vi "main.vi"() -> ()   [LabVIEW 2026]
panel:
  out "Tab Value":T1(ring)
  in  "Error In":errorcluster
  out "Value":T1(ring)
  in  "Tab Control":T1(tab)
  out "pull_indicator":bool
  in  "pull_button":bool
  in  "Commit Message":string
  out "String":string
  in  "commit _button":bool
  out "commit_indicator":bool
  out "git commit output":string
  in  "add_all_button":bool
  out "add_all_indicator":bool
  out "git add output":string
  in  "push_button":bool
  out "push_indicator":bool
  out "git push output":string
  in  "commit message":string
  in  "working directory":path=path ""
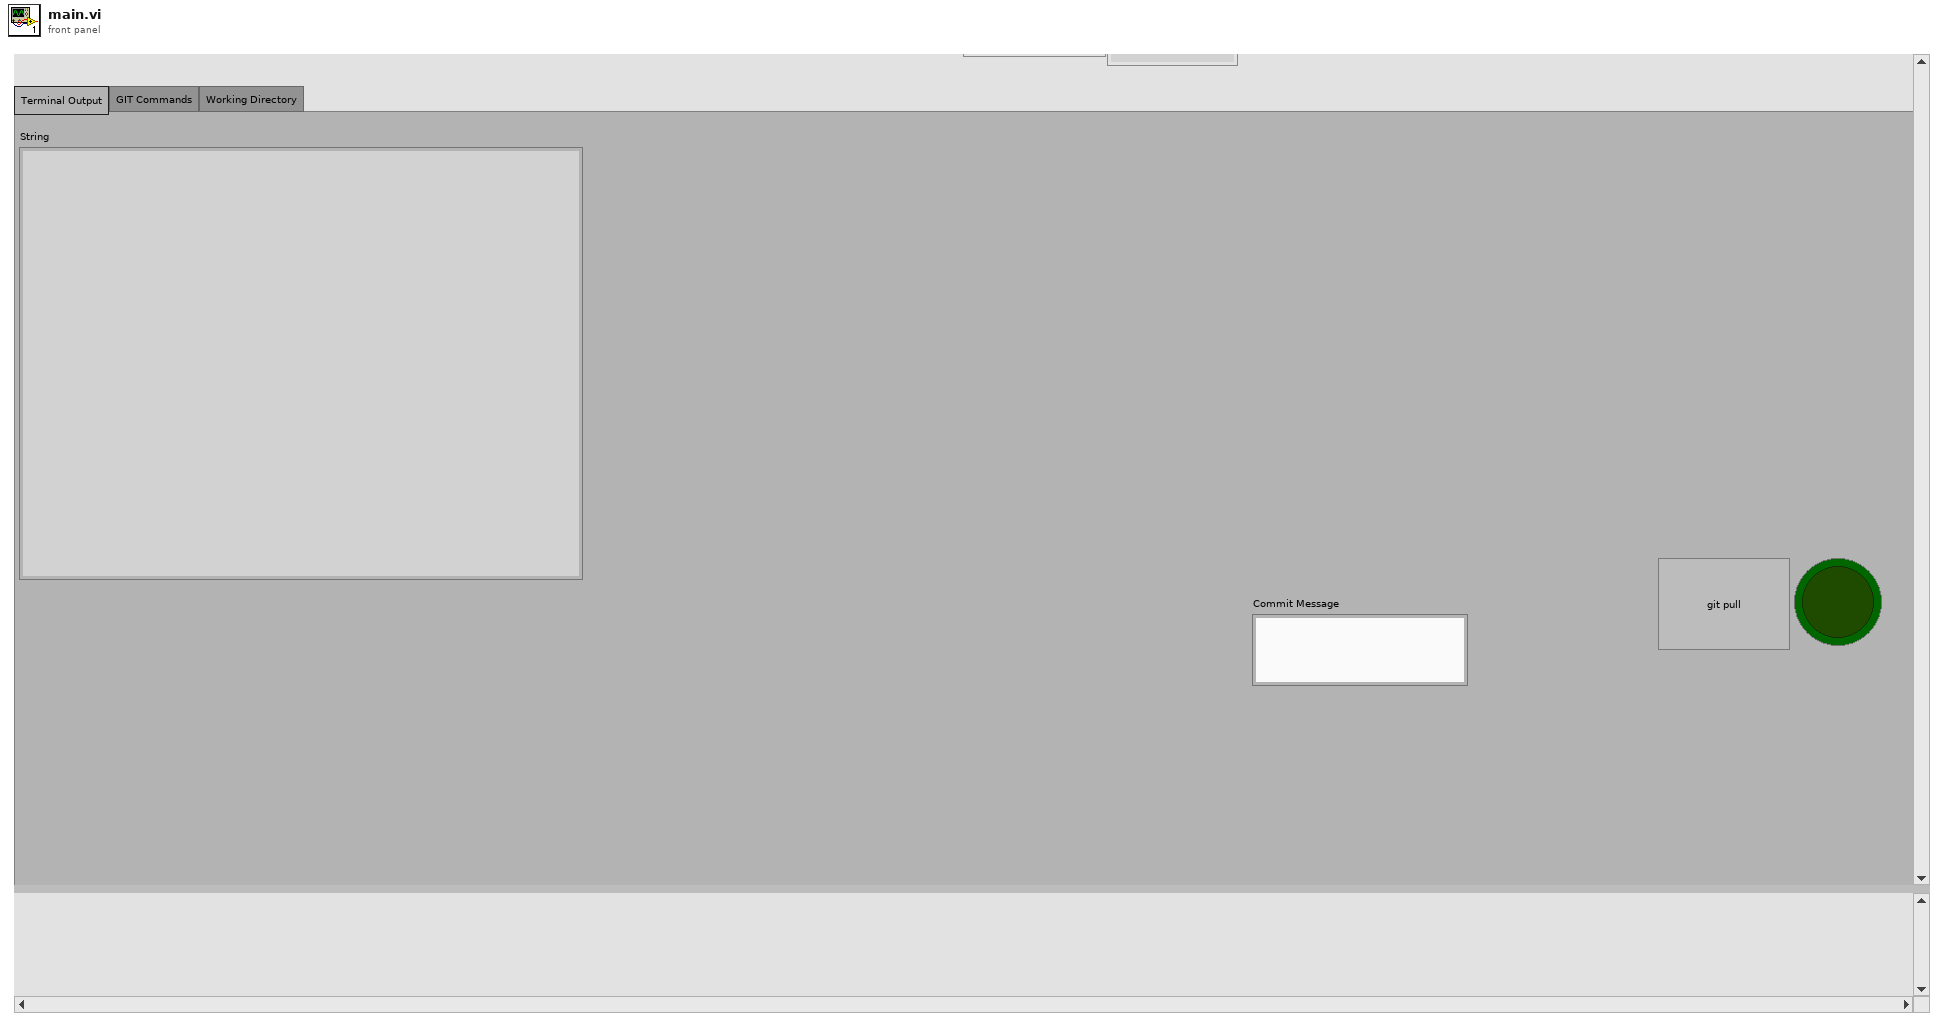
[diagram p1: front panel]
types:
  T1 = enum32{"Terminal Output", "GIT Commands", "Working Directory"}
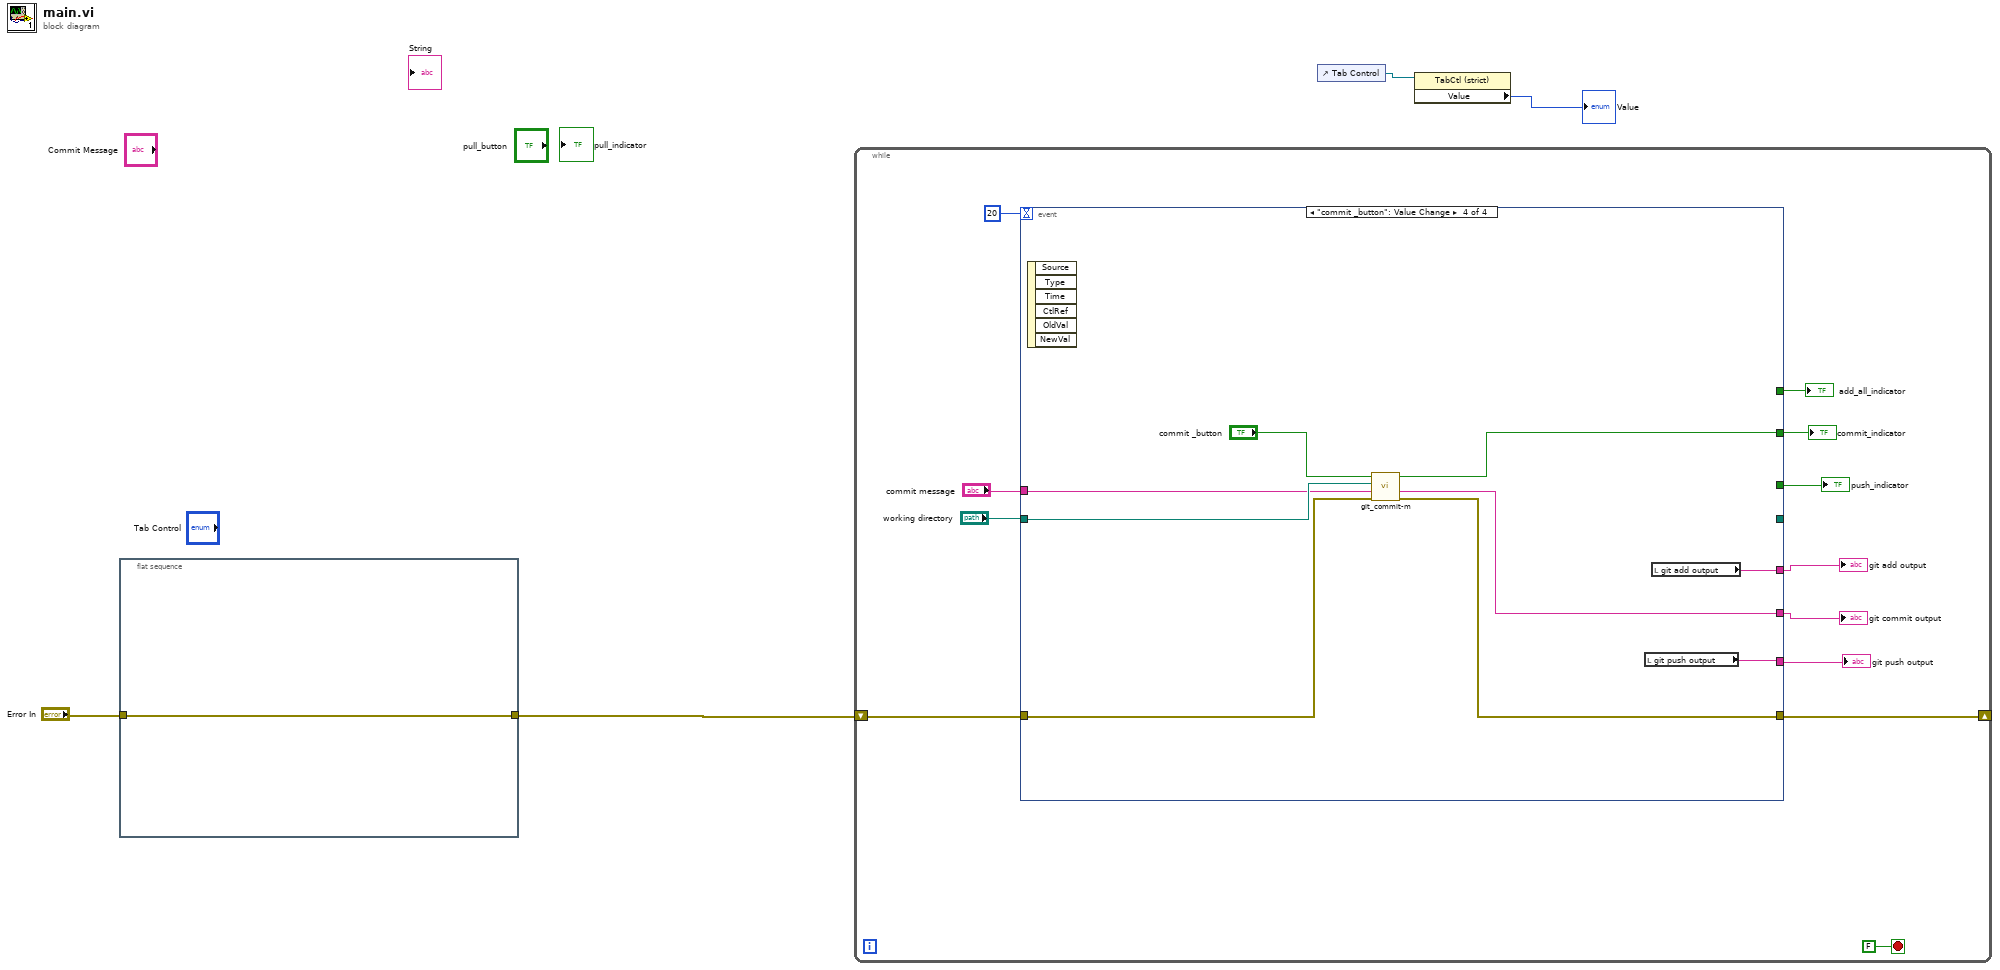
[diagram p0: block diagram]
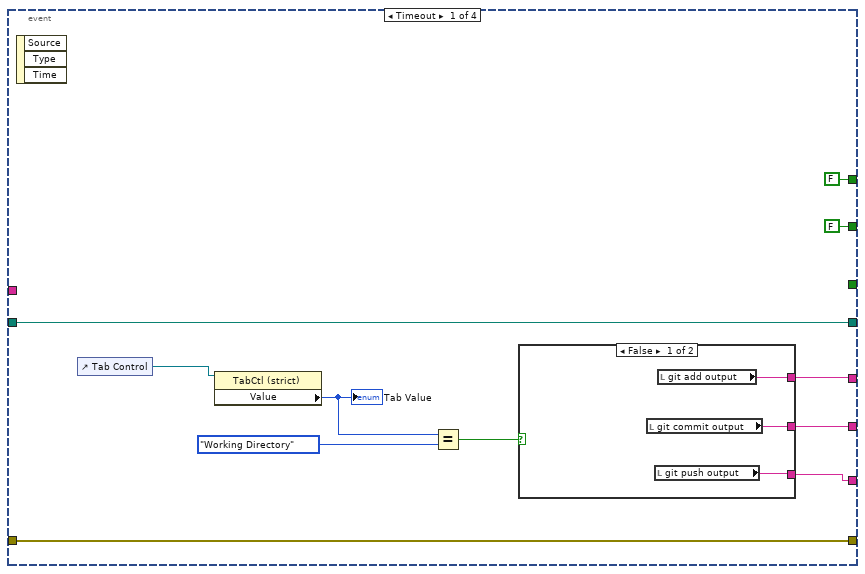
[diagram p2: hidden frame]
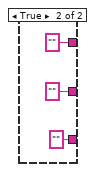
[diagram p3: hidden frame]
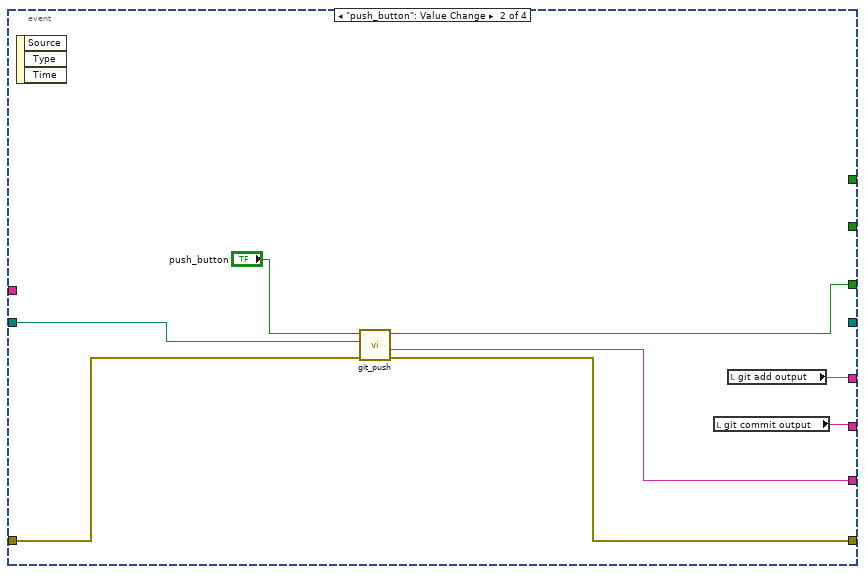
[diagram p4: hidden frame]
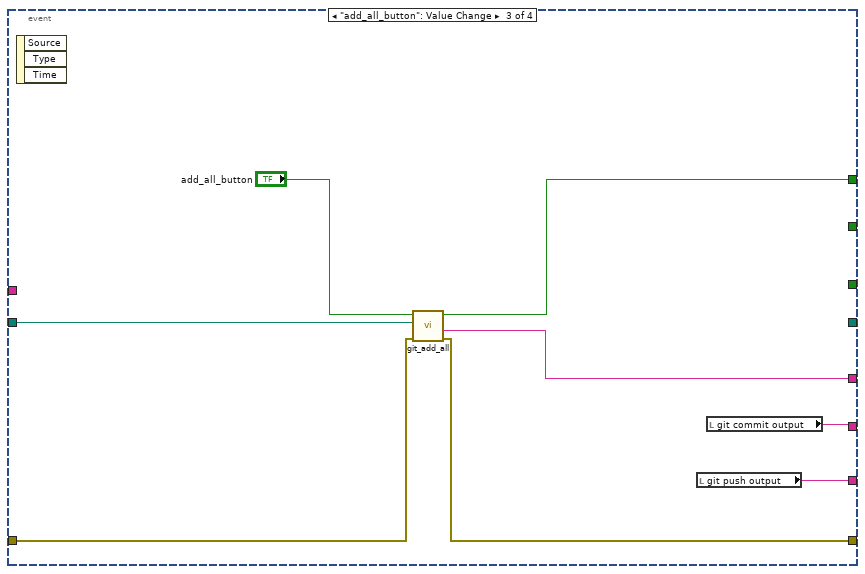
[diagram p5: hidden frame]
diagram:
  n1 = flat-sequence {
    tunnel: [w5] -> w2
    tunnel: "Error In" -> [w5]
    frame #0 {
    }
  }
  n2 = while {
    shift-right: [w14] -> _
    shift-left: w2 -> [w15]
    stop <- FALSE stop-if-true
    n3 = event shown="[3] \"commit _button\": Value Change" {
      selector: _ -> [_ _ _ _]
      dyn-events: _ -> [_ _ _ _]
      timeout: 20 -> [_ _ _ _]
      tunnel: w15 -> [w25 w42 w50 w58]
      tunnel: [w25 w41 w49 w57] -> w14
      tunnel: [FALSE ("add_all_button") _ w46 _] -> w13
      tunnel: "working directory" -> [w26 w37 w47 w56]
      tunnel: [w26 _ _ _] -> _
      tunnel: [FALSE ("commit_indicator") _ _ w55] -> w12
      tunnel: [w23 w36 w44 w54] -> w10
      tunnel: [w24 w35 w45 w53] -> w11
      tunnel: [_ w39 _ _] -> w8
      tunnel: [w18 w40 w43 w52] -> w7
      tunnel: "commit message" -> [_ _ _ w51]
      event Timeout {
        n4 = event-data() -> ()  [unwired: 1 in, 3 out]
        n5 = control-ref of="Tab Control"() -> (w22:refnum<vi>)
        n6 = property class="TabCtl (strict)"(reference=w22) -> ("Value"=w21:T1)  [unwired: 1 in, 2 out]
        "Tab Value" <- w21
        n7 = Equal?(x=w21, y=T1."Working Directory") -> (x = y?=w19:bool)
        n8 = case shown="False" w19 {
          tunnel: [w31 "" ("git add output")] -> w24
          tunnel: [w30 "" ("git commit output")] -> w23
          tunnel: [w29 "" ("git push output")] -> w18
          frame False {
            n9 = local read "git commit output"() -> (w30:string)
            n10 = local read "git push output"() -> (w29:string)
            n11 = local read "git add output"() -> (w31:string)
          }
          frame True {
          }
        }
      }
      event "push_button": Value Change {
        n12 = event-data() -> ()  [unwired: 1 in, 3 out]
        n13 = call "git_push.vi"("Error In"=w42, "Working Directory In"=w37, "push_button"="push_button") -> ("Error Out"=w41:errorcluster, "git push output"=w40:string, "push_indicator"=w39:bool)  [unwired: 5 in, 1 out]
        n14 = local read "git commit output"() -> (w36:string)
        n15 = local read "git add output"() -> (w35:string)
      }
      event "add_all_button": Value Change {
        n16 = event-data() -> ()  [unwired: 1 in, 3 out]
        n17 = call "git_add_all.vi"("Error In"=w50, "Working Directory In"=w47, "add_all_button"="add_all_button") -> ("Error Out"=w49:errorcluster, "git add output"=w45:string, "add_all_indicator"=w46:bool)  [unwired: 5 in, 1 out]
        n18 = local read "git push output"() -> (w43:string)
        n19 = local read "git commit output"() -> (w44:string)
      }
      event "commit _button": Value Change {
        n20 = event-data() -> ()  [unwired: 1 in, 6 out]
        n21 = call "git_commit-m.vi"("Error In"=w58, "commit message"=w51, "Working Directory In"=w56, "commit_button"="commit _button") -> ("Error Out"=w57:errorcluster, "git commit output"=w54:string, "commit_indicator"=w55:bool)  [unwired: 4 in, 1 out]
        n22 = local read "git push output"() -> (w52:string)
        n23 = local read "git add output"() -> (w53:string)
      }
    }
    "add_all_indicator" <- w13
    "commit_indicator" <- w12
    "git commit output" <- w10
    "git add output" <- w11
    "push_indicator" <- w8
    "git push output" <- w7
  }
  n24 = control-ref of="Tab Control"() -> (w4:refnum<vi>)
  n25 = property class="TabCtl (strict)"(reference=w4) -> ("Value"=→"Value":T1)  [unwired: 1 in, 2 out]
